vi "AutonIndexLoad.vi"() -> (0 "index":i32)   [LabVIEW 2013]
uses:
  <vilib>/Utility/config.llb/Read Key (I32).vi
  <vilib>/Utility/config.llb/NI_LVConfig.lvlib
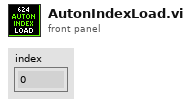
[diagram p1: front panel]
types:
  T1 = typedef "NI_LVConfig.lvlib/Config Data RefNum.ctl" = refnum<k1>
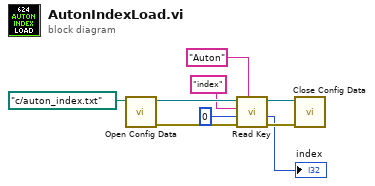
[diagram p0: block diagram]
diagram:
  n1 = call <vilib>:"Open Config Data.vi"("configuration file path"=path "c:/auton_index.txt") -> ("error out"=w3:errorcluster, "refnum"=w8:T1)  [unwired: 8 in, 1 out]
  n2 = call-poly <vilib>:"Read Key.vi"("section"="Auton", "error in (no error)"=w3, "default value"=0, "key"="index", "refnum"=w8) -> ("error out"=w5:errorcluster, "value"=→"index":i32, "refnum out"=w4:T1)  [unwired: 3 in, 1 out]
  n3 = call <vilib>:"Close Config Data.vi"("error in (no error)"=w5, "refnum"=w4) -> ()  [unwired: 8 in, 2 out]
